vi "Dual_Joy_Ctrl.vi"(8 "Joy1_0(X)":dbl, 9 "Joy1_1(Y)":dbl, 10 "Joy0_0(X)":dbl, 11 "Joy0_1(Y)":dbl) -> (1 "Z":dbl, 2 "Y":dbl, 3 "X":dbl)   [LabVIEW 2017]
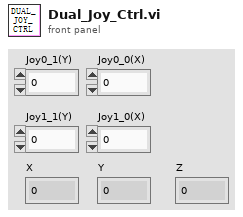
[diagram p1: front panel]
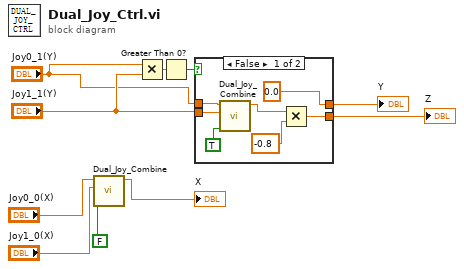
[diagram p0: block diagram]
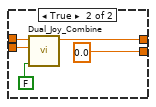
[diagram p2: hidden frame]
diagram:
  n1 = call "Dual_Joy_Combine.vi"("Joy1"="Joy0_0(X)", "Joy2"="Joy1_0(X)", "Z"=FALSE) -> ("Output"=→"X":dbl)  [unwired: 7 in]
  n2 = Multiply(x="Joy0_1(Y)", y="Joy1_1(Y)") -> (x*y=w5:dbl)
  n3 = Greater Than 0?(x=w5) -> (x > 0?=w6:bool)
  n4 = case shown="False" w6 {
    tunnel: "Joy1_1(Y)" -> [w13 w22]
    tunnel: "Joy0_1(Y)" -> [w14 w21]
    tunnel: [0.0 w20] -> w4
    tunnel: [w16 0.0] -> w3
    frame False {
      n5 = call "Dual_Joy_Combine.vi"("Joy1"=w14, "Joy2"=w13, "Z"=TRUE) -> ("Output"=w12:dbl)  [unwired: 7 in]
      n6 = Multiply(x=w12, y=-0.8) -> (x*y=w16:dbl)
    }
    frame True {
      n7 = call "Dual_Joy_Combine.vi"("Joy1"=w21, "Joy2"=w22, "Z"=FALSE) -> ("Output"=w20:dbl)  [unwired: 7 in]
    }
  }
  "Y" <- w4
  "Z" <- w3
